vi "UI Selection Valve.vi"(8 "error in":errorcluster) -> (0 "error out":errorcluster)   [LabVIEW 2019, in "Test.lvlib"]
uses:
  Test.lvlib
  Fluidic Process/SubVI/Fluidic Para.ctl
  <vilib>/Utility/file.llb/Read Delimited Spreadsheet (string).vi
  Controller/Controller.lvlib
  Queues/Queues.lvlib
  Fluidic Process/Fluidic Process.lvlib
panel:
  in  "Purge":bool
  in  "Flow Rate":bool
  in  "Stop Process":bool
  out "Remaining Time(s)":dbl
  out "Total Process":string
  out "Current Process":string
  out "Gauge":dbl(knob)=1.2869315802184793e-48 scale=0.0..100.0
  in  "Selection Valve Hold Pressure":bool
  in  "Chip Hold Pressure":bool
  in  "Back":bool
  # "/"
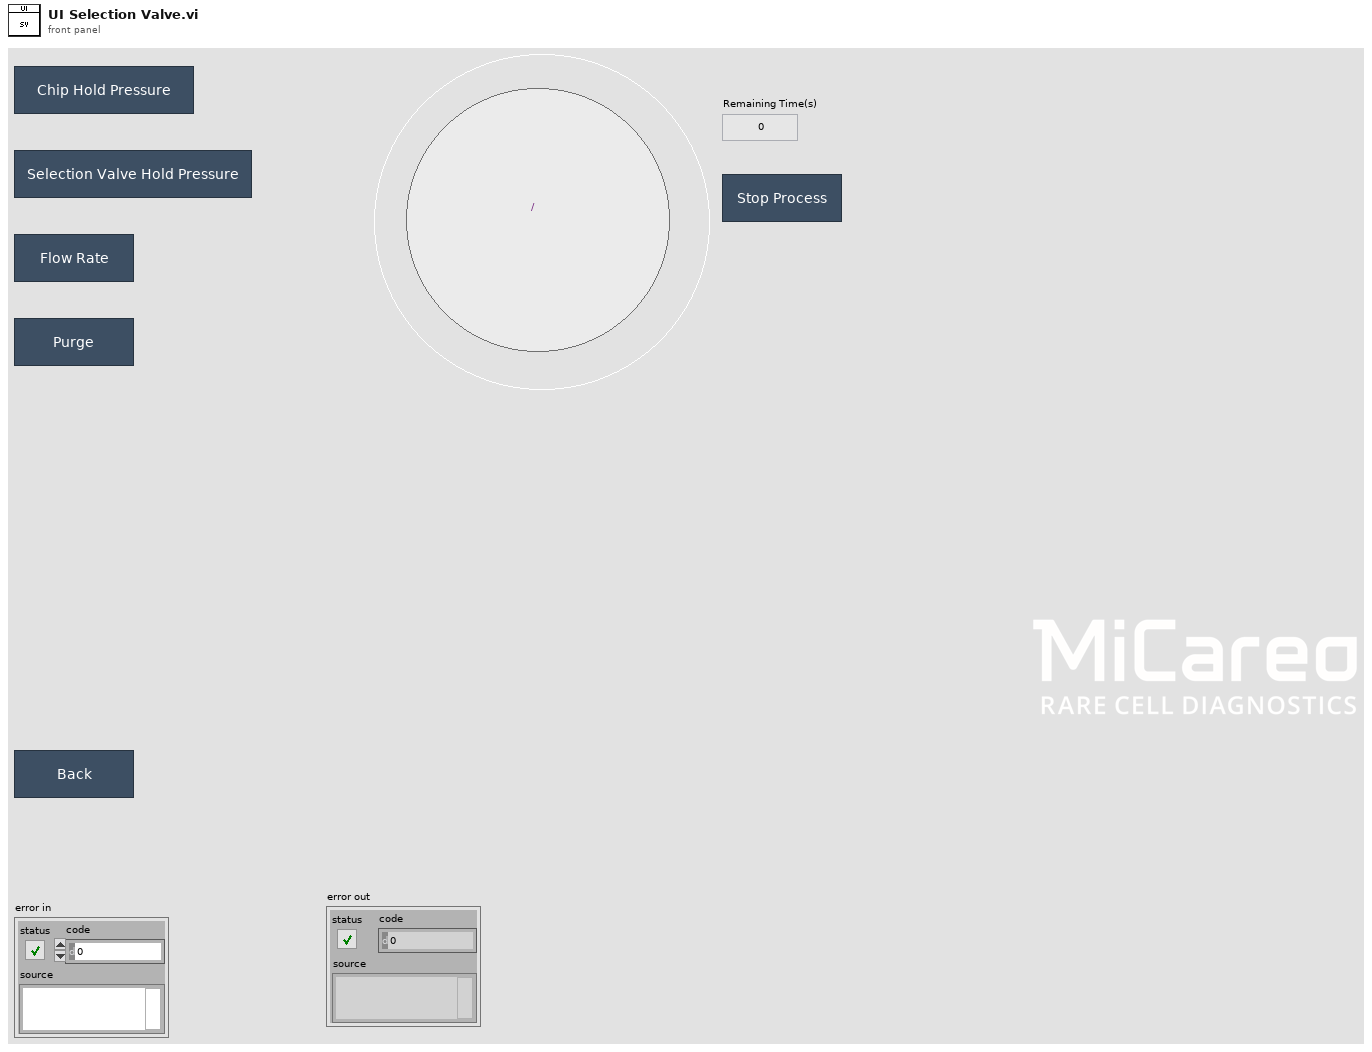
[diagram p1: front panel]
types:
  T1 = enum8{"Enabled", "Disabled", "Disabled and Grayed Out"}
  T2 = typedef "Fluidic Process.lvlib/Fluidic Para.ctl" = cluster{"Read Force Sensor":i32, "Read Regulator":i32, "Read Force Sensor?":bool, "Read Regulator?":bool, "Read Syringe Pump":i32, "Read Syringe Pump?":bool}
  T3 = typedef "Fluidic Process.lvlib/SEQ Data.ctl" = cluster{"Fluidic Process Done?":bool, "Current Process":i32, "Remaining Time":dbl, "Total Process":i32, "Air Sealing":bool, "Force Condition":bool}
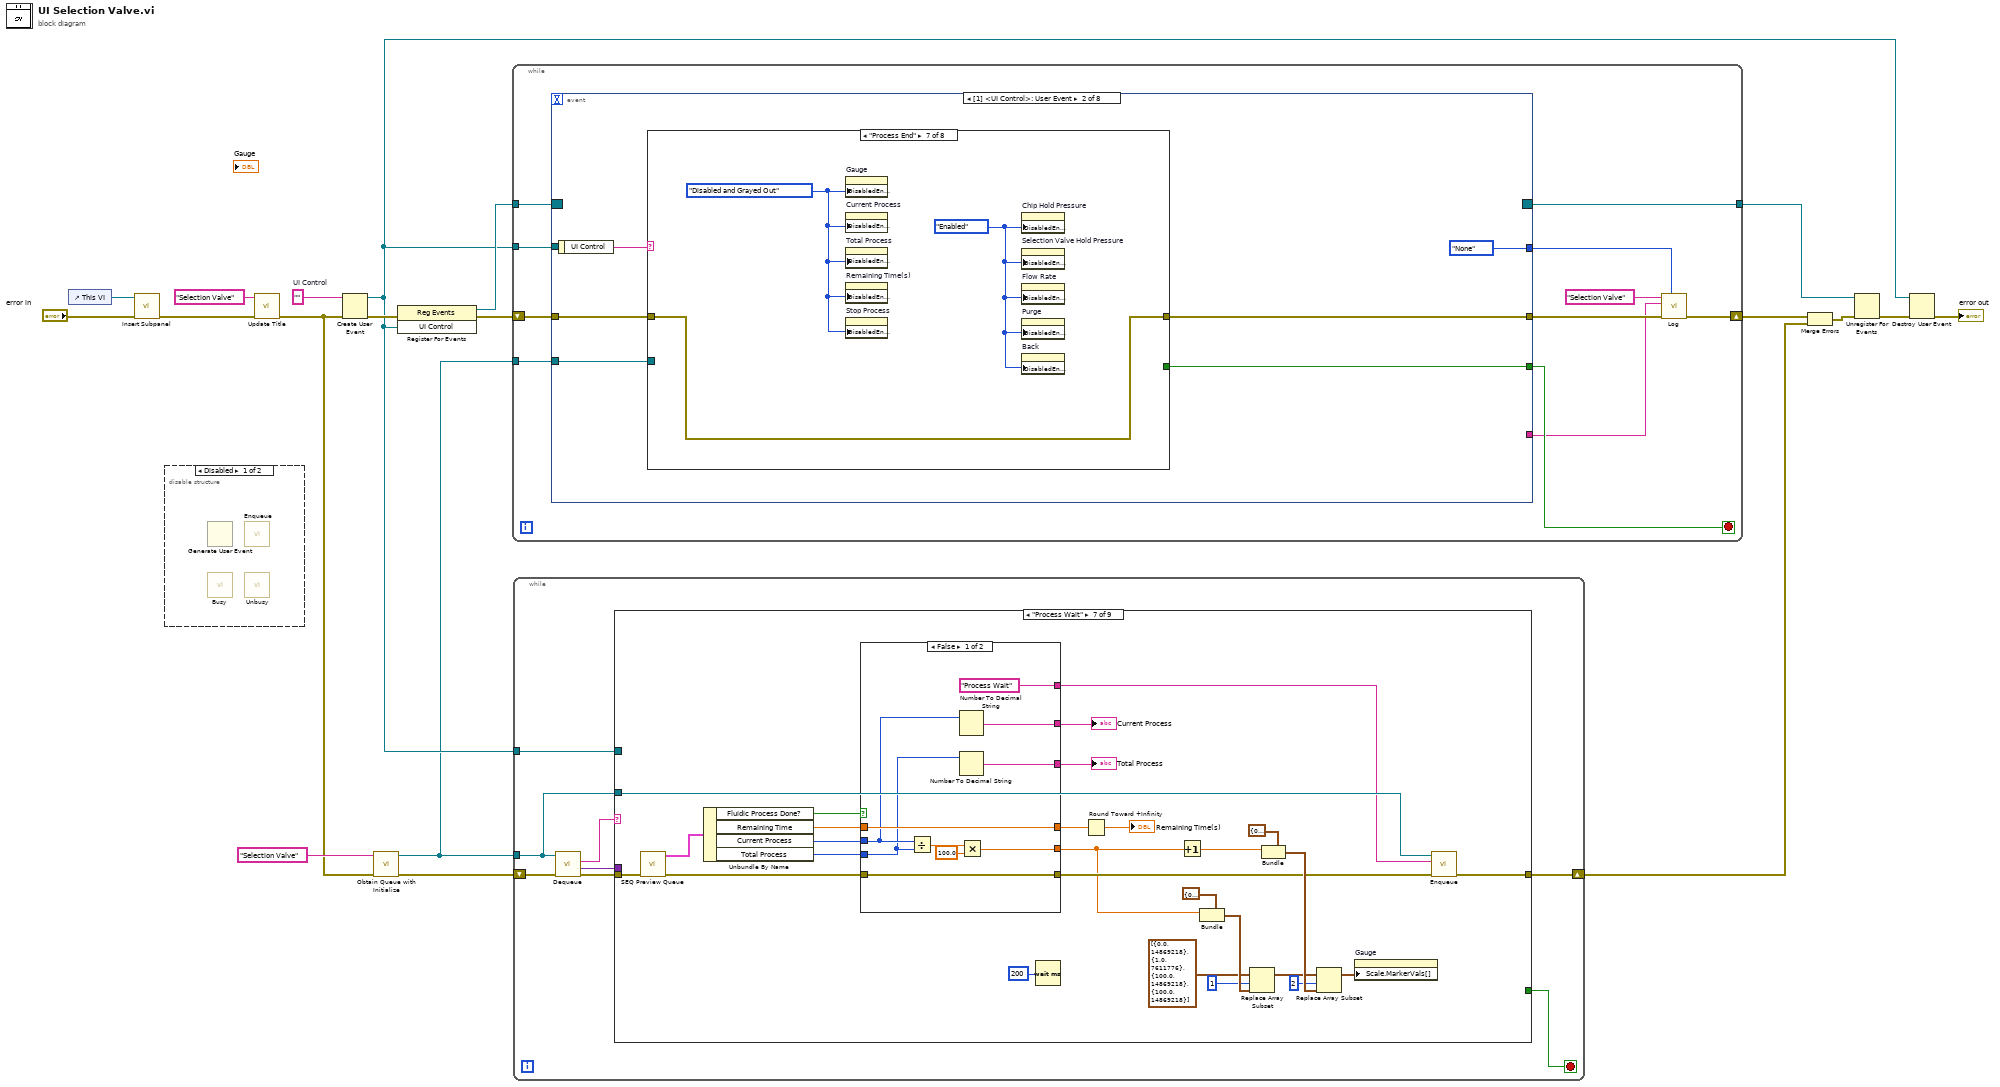
[diagram p0: block diagram]
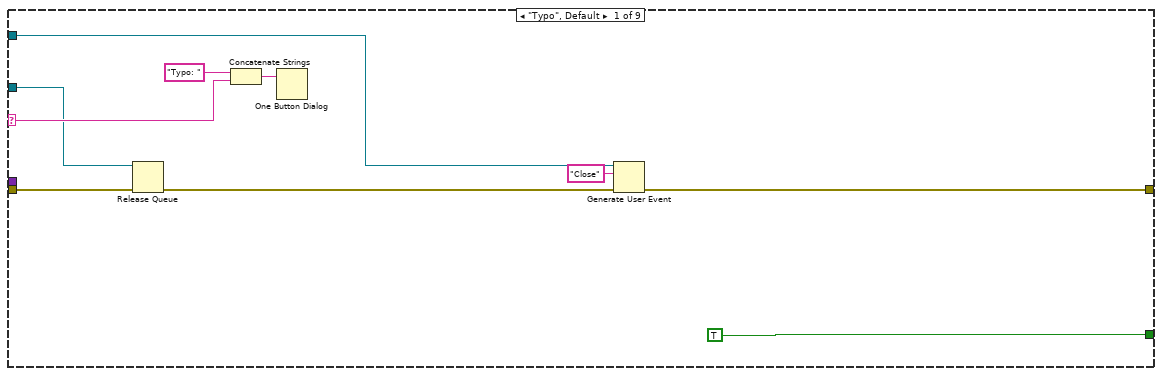
[diagram p3: hidden frame]
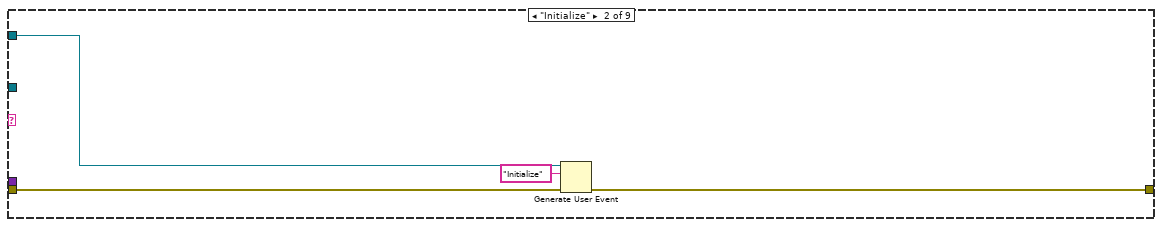
[diagram p4: hidden frame]
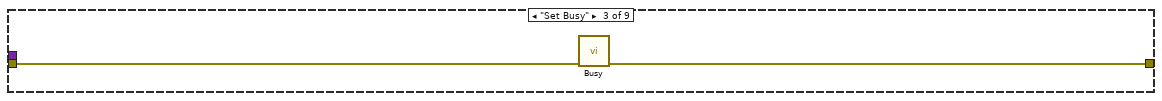
[diagram p5: hidden frame]
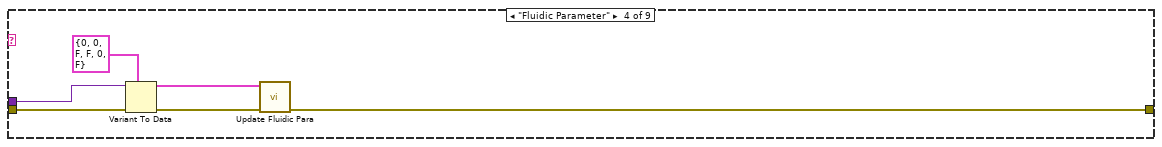
[diagram p6: hidden frame]
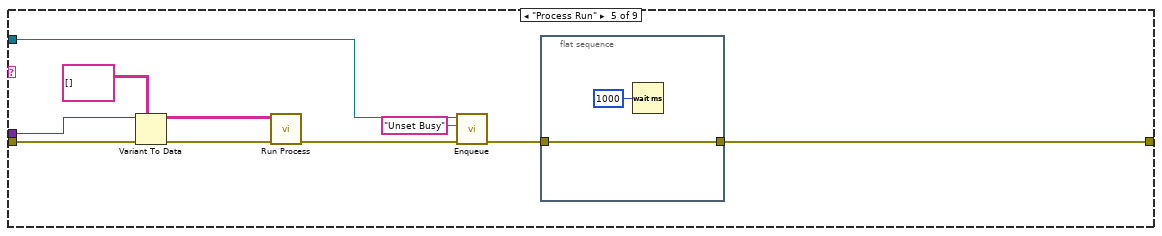
[diagram p7: hidden frame]
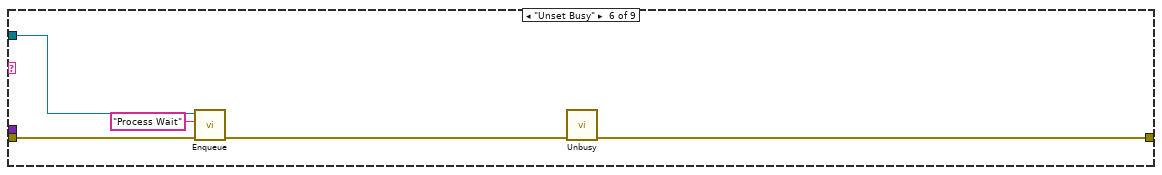
[diagram p8: hidden frame]
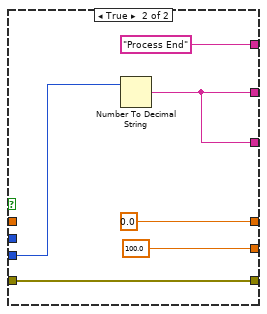
[diagram p9: hidden frame]
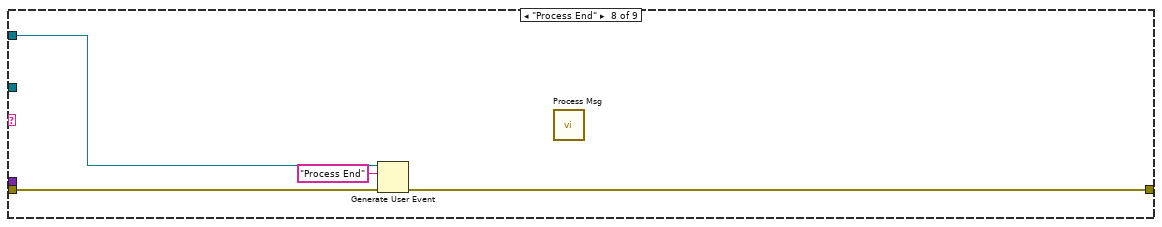
[diagram p10: hidden frame]
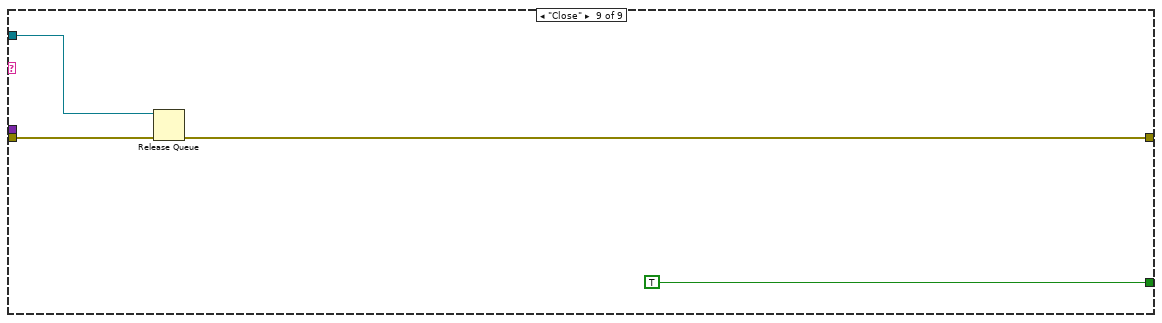
[diagram p11: hidden frame]
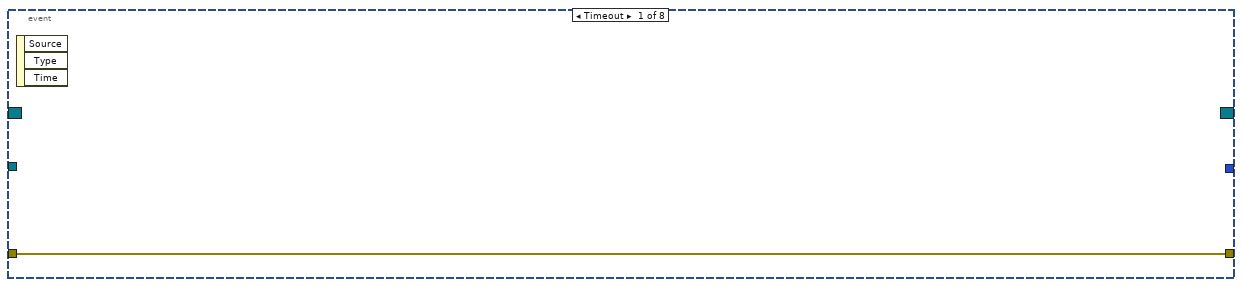
[diagram p12: hidden frame]
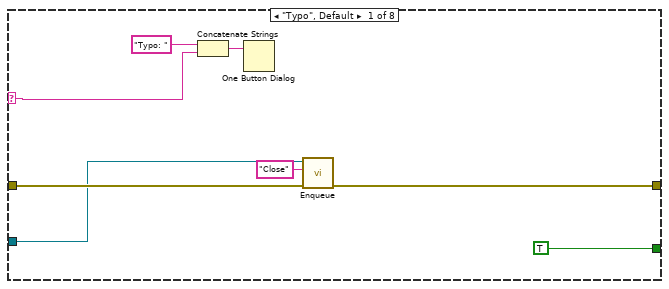
[diagram p13: hidden frame]
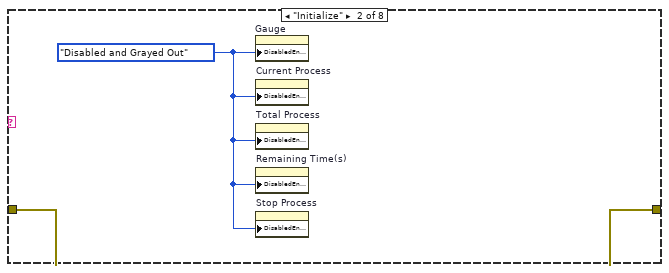
[diagram p14: hidden frame]
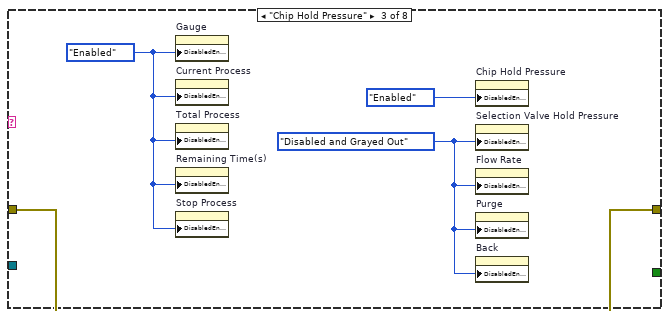
[diagram p15: hidden frame]
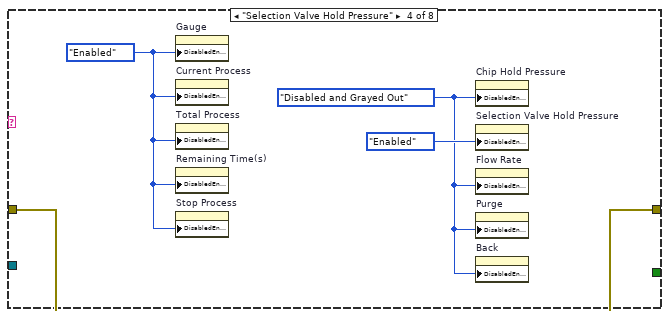
[diagram p16: hidden frame]
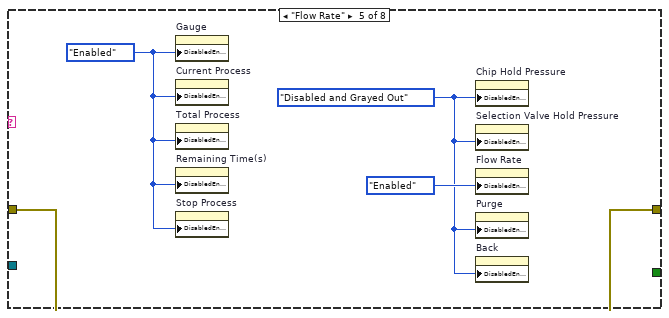
[diagram p17: hidden frame]
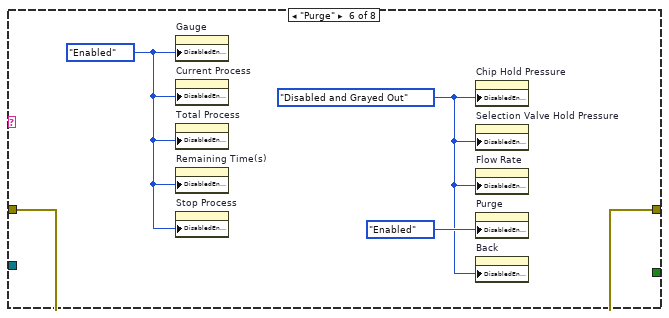
[diagram p18: hidden frame]
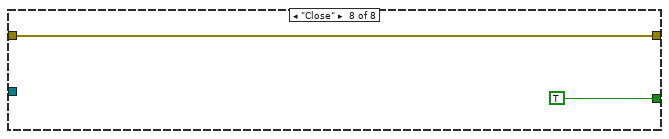
[diagram p19: hidden frame]
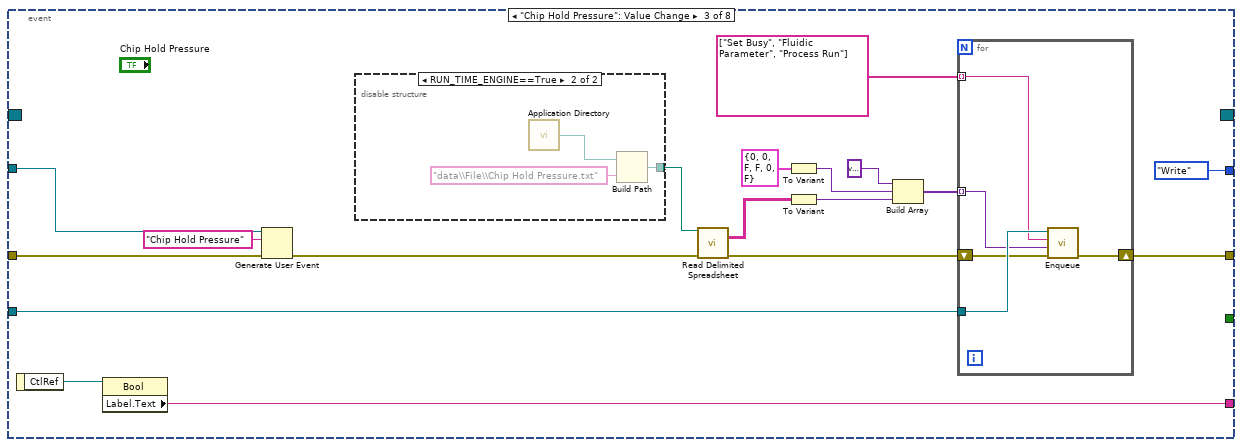
[diagram p20: hidden frame]
diagram:
  w9 = ""  # UI Control
  n1 = control-ref of="This VI"() -> (w8:refnum<vi>)
  n2 = call "Insert Subpanel.vi"("Error In"="error in", "VI Refnum"=w8) -> ("Error Out"=w3:errorcluster)  [unwired: 9 in]
  n3 = disable-structure shown="Disabled" {
    frame Disabled {
      n4 = Generate User Event() -> ()  [unwired: 4 in, 2 out]
      n5 = call "Busy.vi"() -> ()  [unwired: 11 in, 1 out]
      n6 = call "Enqueue.vi"() -> ()  [unwired: 10 in, 2 out]
      n7 = call "Unbusy.vi"() -> ()  [unwired: 11 in, 1 out]
    }
    frame Enabled {
    }
  }
  n8 = call "Update Title.vi"("Error In"=w3, "Title"="Selection Valve") -> ("Error Out"=w2:errorcluster)  [unwired: 9 in]
  n9 = Create User Event(user event datatype=w9, error in=w2) -> (user event=w7:refnum<user-event>, error out=w18:errorcluster)
  n10 = call "Obtain Queue with Initialize.vi"("Error In"=w2, "Queue Name"="Selection Valve") -> ("Error Out"=w6:errorcluster, "Queue out"=w5:refnum<queue>)  [unwired: 8 in]
  n11 = register-events(error in=w18, w7) -> (reference out=w16:refnum<event-registration>, error out=w17:errorcluster)  [unwired: 1 in]
  n12 = while {
    tunnel: w16 -> [w28]
    tunnel: w5 -> [w27]
    shift-right: [w23] -> w14
    shift-left: w17 -> [w30]
    tunnel: [w26] -> w12
    tunnel: w7 -> [w25]
    stop <- w29 stop-if-true
    n13 = event shown="[1] <UI Control>: User Event" {
      selector: w28 -> [_ _ _ _ _ _ _ _]
      dyn-events: [_ _ _ _ _ _ _ _] -> w26
      timeout: _ -> [_ _ _ _ _ _ _ _]
      tunnel: w30 -> [w31 w37 w75 w104 w133 w162 w189 w193]
      tunnel: [_ w33 _ _ _ _ _ TRUE] -> w29
      tunnel: w27 -> [_ w35 w86 w115 w144 w173 _ w195]
      tunnel: [w31 w34 w82 w111 w140 w169 w188 w196] -> w24
      tunnel: w25 -> [_ _ w73 w102 w131 w160 _ _]
      tunnel: [_ enum16{"None", "Write"}."None" ("Action") enum16{"None", "Write"}."Write" ("Action") enum16{"None", "Write"}."Write" ("Action") enum16{"None", "Write"}."Write" ("Action") enum16{"None", "Write"}."Write" ("Action") enum16{"None", "Write"}."Write" ("Action") enum16{"None", "Write"}."Write" ("Action")] -> w21
      tunnel: [_ _ w70 w98 w127 w156 w185 w190] -> w20
      event Timeout {
        n14 = event-data() -> ()  [unwired: 1 in, 3 out]
      }
      event User Event {
        n15 = event-data() -> ("UI Control"=w36:string)  [unwired: 1 in]
        n16 = case shown="\"Process End\"" w36 {
          selector: w36 -> [w40 _ _ _ _ _ _ _]
          tunnel: w37 -> [w45 w47 w51 w55 w59 w63 w66 w68]
          tunnel: w35 -> [w44 _ _ _ _ _ _ _]
          tunnel: [w39 w47 w51 w55 w59 w63 w66 w68] -> w34
          tunnel: [TRUE _ _ _ _ _ _ TRUE] -> w33
          frame "Typo", Default {
            n17 = Concatenate Strings("Typo: " ("string"), w40) -> (w41:string)
            n18 = One Button Dialog(message=w41) -> ()  [unwired: 1 in, 1 out]
            n19 = call "Enqueue.vi"("Error In"=w45, "State"="Close", "Queue in"=w44) -> ("Error Out"=w39:errorcluster)  [unwired: 7 in, 1 out]
          }
          frame "Initialize" {
            w46 = T1."Disabled and Grayed Out" ("Disabled")
            n20 = property on="Gauge" class="Knob (strict)"("DisabledEnum"=w46) -> ()  [unwired: 2 in, 2 out]
            n21 = property on="Current Process" class="Str"("DisabledEnum"=w46) -> ()  [unwired: 2 in, 2 out]
            n22 = property on="Total Process" class="Str"("DisabledEnum"=w46) -> ()  [unwired: 2 in, 2 out]
            n23 = property on="Remaining Time(s)" class="DigNum (strict)"("DisabledEnum"=w46) -> ()  [unwired: 2 in, 2 out]
            n24 = property on="Stop Process" class="Bool"("DisabledEnum"=w46) -> ()  [unwired: 2 in, 2 out]
          }
          frame "Chip Hold Pressure" {
            w49 = T1."Enabled" ("Disabled")
            w48 = T1."Disabled and Grayed Out" ("Disabled")
            n25 = property on="Gauge" class="Knob (strict)"("DisabledEnum"=w49) -> ()  [unwired: 2 in, 2 out]
            n26 = property on="Current Process" class="Str"("DisabledEnum"=w49) -> ()  [unwired: 2 in, 2 out]
            n27 = property on="Total Process" class="Str"("DisabledEnum"=w49) -> ()  [unwired: 2 in, 2 out]
            n28 = property on="Remaining Time(s)" class="DigNum (strict)"("DisabledEnum"=w49) -> ()  [unwired: 2 in, 2 out]
            n29 = property on="Stop Process" class="Bool"("DisabledEnum"=w49) -> ()  [unwired: 2 in, 2 out]
            n30 = property on="Chip Hold Pressure" class="Bool"("DisabledEnum"=T1."Enabled" ("Disabled")) -> ()  [unwired: 2 in, 2 out]
            n31 = property on="Selection Valve Hold Pressure" class="Bool"("DisabledEnum"=w48) -> ()  [unwired: 2 in, 2 out]
            n32 = property on="Flow Rate" class="Bool"("DisabledEnum"=w48) -> ()  [unwired: 2 in, 2 out]
            n33 = property on="Purge" class="Bool"("DisabledEnum"=w48) -> ()  [unwired: 2 in, 2 out]
            n34 = property on="Back" class="Bool"("DisabledEnum"=w48) -> ()  [unwired: 2 in, 2 out]
          }
          frame "Selection Valve Hold Pressure" {
            w54 = T1."Enabled" ("Disabled")
            w52 = T1."Disabled and Grayed Out" ("Disabled")
            n35 = property on="Gauge" class="Knob (strict)"("DisabledEnum"=w54) -> ()  [unwired: 2 in, 2 out]
            n36 = property on="Current Process" class="Str"("DisabledEnum"=w54) -> ()  [unwired: 2 in, 2 out]
            n37 = property on="Total Process" class="Str"("DisabledEnum"=w54) -> ()  [unwired: 2 in, 2 out]
            n38 = property on="Remaining Time(s)" class="DigNum (strict)"("DisabledEnum"=w54) -> ()  [unwired: 2 in, 2 out]
            n39 = property on="Stop Process" class="Bool"("DisabledEnum"=w54) -> ()  [unwired: 2 in, 2 out]
            n40 = property on="Chip Hold Pressure" class="Bool"("DisabledEnum"=w52) -> ()  [unwired: 2 in, 2 out]
            n41 = property on="Selection Valve Hold Pressure" class="Bool"("DisabledEnum"=T1."Enabled" ("Disabled")) -> ()  [unwired: 2 in, 2 out]
            n42 = property on="Flow Rate" class="Bool"("DisabledEnum"=w52) -> ()  [unwired: 2 in, 2 out]
            n43 = property on="Purge" class="Bool"("DisabledEnum"=w52) -> ()  [unwired: 2 in, 2 out]
            n44 = property on="Back" class="Bool"("DisabledEnum"=w52) -> ()  [unwired: 2 in, 2 out]
          }
          frame "Flow Rate" {
            w58 = T1."Enabled" ("Disabled")
            w56 = T1."Disabled and Grayed Out" ("Disabled")
            n45 = property on="Gauge" class="Knob (strict)"("DisabledEnum"=w58) -> ()  [unwired: 2 in, 2 out]
            n46 = property on="Current Process" class="Str"("DisabledEnum"=w58) -> ()  [unwired: 2 in, 2 out]
            n47 = property on="Total Process" class="Str"("DisabledEnum"=w58) -> ()  [unwired: 2 in, 2 out]
            n48 = property on="Remaining Time(s)" class="DigNum (strict)"("DisabledEnum"=w58) -> ()  [unwired: 2 in, 2 out]
            n49 = property on="Stop Process" class="Bool"("DisabledEnum"=w58) -> ()  [unwired: 2 in, 2 out]
            n50 = property on="Chip Hold Pressure" class="Bool"("DisabledEnum"=w56) -> ()  [unwired: 2 in, 2 out]
            n51 = property on="Selection Valve Hold Pressure" class="Bool"("DisabledEnum"=w56) -> ()  [unwired: 2 in, 2 out]
            n52 = property on="Flow Rate" class="Bool"("DisabledEnum"=T1."Enabled" ("Disabled")) -> ()  [unwired: 2 in, 2 out]
            n53 = property on="Purge" class="Bool"("DisabledEnum"=w56) -> ()  [unwired: 2 in, 2 out]
            n54 = property on="Back" class="Bool"("DisabledEnum"=w56) -> ()  [unwired: 2 in, 2 out]
          }
          frame "Purge" {
            w62 = T1."Enabled" ("Disabled")
            w60 = T1."Disabled and Grayed Out" ("Disabled")
            n55 = property on="Gauge" class="Knob (strict)"("DisabledEnum"=w62) -> ()  [unwired: 2 in, 2 out]
            n56 = property on="Current Process" class="Str"("DisabledEnum"=w62) -> ()  [unwired: 2 in, 2 out]
            n57 = property on="Total Process" class="Str"("DisabledEnum"=w62) -> ()  [unwired: 2 in, 2 out]
            n58 = property on="Remaining Time(s)" class="DigNum (strict)"("DisabledEnum"=w62) -> ()  [unwired: 2 in, 2 out]
            n59 = property on="Stop Process" class="Bool"("DisabledEnum"=w62) -> ()  [unwired: 2 in, 2 out]
            n60 = property on="Chip Hold Pressure" class="Bool"("DisabledEnum"=w60) -> ()  [unwired: 2 in, 2 out]
            n61 = property on="Selection Valve Hold Pressure" class="Bool"("DisabledEnum"=w60) -> ()  [unwired: 2 in, 2 out]
            n62 = property on="Flow Rate" class="Bool"("DisabledEnum"=w60) -> ()  [unwired: 2 in, 2 out]
            n63 = property on="Purge" class="Bool"("DisabledEnum"=T1."Enabled" ("Disabled")) -> ()  [unwired: 2 in, 2 out]
            n64 = property on="Back" class="Bool"("DisabledEnum"=w60) -> ()  [unwired: 2 in, 2 out]
          }
          frame "Process End" {
            w65 = T1."Disabled and Grayed Out" ("Disabled")
            w64 = T1."Enabled" ("Disabled")
            n65 = property on="Gauge" class="Knob (strict)"("DisabledEnum"=w65) -> ()  [unwired: 2 in, 2 out]
            n66 = property on="Current Process" class="Str"("DisabledEnum"=w65) -> ()  [unwired: 2 in, 2 out]
            n67 = property on="Total Process" class="Str"("DisabledEnum"=w65) -> ()  [unwired: 2 in, 2 out]
            n68 = property on="Remaining Time(s)" class="DigNum (strict)"("DisabledEnum"=w65) -> ()  [unwired: 2 in, 2 out]
            n69 = property on="Stop Process" class="Bool"("DisabledEnum"=w65) -> ()  [unwired: 2 in, 2 out]
            n70 = property on="Chip Hold Pressure" class="Bool"("DisabledEnum"=w64) -> ()  [unwired: 2 in, 2 out]
            n71 = property on="Selection Valve Hold Pressure" class="Bool"("DisabledEnum"=w64) -> ()  [unwired: 2 in, 2 out]
            n72 = property on="Flow Rate" class="Bool"("DisabledEnum"=w64) -> ()  [unwired: 2 in, 2 out]
            n73 = property on="Purge" class="Bool"("DisabledEnum"=w64) -> ()  [unwired: 2 in, 2 out]
            n74 = property on="Back" class="Bool"("DisabledEnum"=w64) -> ()  [unwired: 2 in, 2 out]
          }
          frame "Close" {
          }
        }
      }
      event "Chip Hold Pressure": Value Change {
        n75 = event-data() -> ("CtlRef"=w71:refnum<vi>)  [unwired: 1 in]
        n76 = property class="Bool"(reference=w71) -> ("Label.Text"=w70:string)  [unwired: 1 in, 2 out]
        n77 = Generate User Event(user event=w73, event data cluster="Chip Hold Pressure" ("event data"), error in=w75) -> (error out=w74:errorcluster)  [unwired: 1 in, 1 out]
        n78 = disable-structure shown="RUN_TIME_ENGINE==True" {
          disable-tunnel: [w87 w90] -> w84
          frame condition #0 (active) {
            n79 = call <vilib>:"Application Directory.vi"() -> ("Application Directory"=w89:path)
            n80 = Build Path(base path=w89, name or relative path="Fluidic Process\\File\\Chip Hold Pressure.txt") -> (appended path=w87:path)
          }
          frame condition #1 {
            n81 = call <vilib>:"Application Directory.vi"() -> ("Application Directory"=w92:path)
            n82 = Build Path(base path=w92, name or relative path="data\\File\\Chip Hold Pressure.txt") -> (appended path=w90:path)
          }
        }
        n83 = call-poly <vilib>:"Read Delimited Spreadsheet.vi"("file path (dialog if empty)"=w84, "error in (no error)"=w74) -> ("all rows"=w83:string[][], "error out"=w85:errorcluster)  [unwired: 8 in, 4 out]
        n84 = To Variant(anything=T2 {"Read Force Sensor"=0, "Read Regulator"=0, "Read Force Sensor?"=FALSE, "Read Regulator?"=FALSE, "Read Syringe Pump"=0, "Read Syringe Pump?"=FALSE} ("Cluster")) -> (Variant=w78:variant)
        n85 = To Variant(anything=w83) -> (Variant=w80:variant)
        n86 = Build Array(variant, w78, w80) -> (w77:variant[])
        n87 = for {
          tunnel: w86 -> [w97]
          shift-right: [w95] -> w82
          shift-left: w85 -> [w96]
          tunnel: string[] ["Set Busy", "Fluidic Parameter", "Process Run"] -> [w94] mode=indexing
          tunnel: w77 -> [w93] mode=indexing
          n88 = call "Enqueue.vi"("Error In"=w96, "Data"=w93, "State"=w94, "Queue in"=w97) -> ("Error Out"=w95:errorcluster)  [unwired: 6 in, 1 out]
        }
      }
      event "Selection Valve Hold Pressure": Value Change {
        n89 = event-data() -> ("CtlRef"=w99:refnum<vi>)  [unwired: 1 in]
        n90 = property class="Bool"(reference=w99) -> ("Label.Text"=w98:string)  [unwired: 1 in, 2 out]
        n91 = Generate User Event(user event=w102, event data cluster="Selection Valve Hold Pressure" ("event data"), error in=w104) -> (error out=w103:errorcluster)  [unwired: 1 in, 1 out]
        n92 = disable-structure shown="RUN_TIME_ENGINE==False, Default" {
          disable-tunnel: [w116 w119] -> w113
          frame condition #0 (active) {
            n93 = call <vilib>:"Application Directory.vi"() -> ("Application Directory"=w118:path)
            n94 = Build Path(base path=w118, name or relative path="Fluidic Process\\File\\Selection Valve Hold Pressure.txt") -> (appended path=w116:path)
          }
          frame condition #1 {
            n95 = call <vilib>:"Application Directory.vi"() -> ("Application Directory"=w121:path)
            n96 = Build Path(base path=w121, name or relative path="data\\File\\Selection Valve Hold Pressure.txt") -> (appended path=w119:path)
          }
        }
        n97 = call-poly <vilib>:"Read Delimited Spreadsheet.vi"("file path (dialog if empty)"=w113, "error in (no error)"=w103) -> ("all rows"=w112:string[][], "error out"=w114:errorcluster)  [unwired: 8 in, 4 out]
        n98 = To Variant(anything=T2 {"Read Force Sensor"=0, "Read Regulator"=0, "Read Force Sensor?"=FALSE, "Read Regulator?"=FALSE, "Read Syringe Pump"=0, "Read Syringe Pump?"=FALSE} ("Cluster")) -> (Variant=w107:variant)
        n99 = To Variant(anything=w112) -> (Variant=w109:variant)
        n100 = Build Array(variant, w107, w109) -> (w106:variant[])
        n101 = for {
          tunnel: w115 -> [w126]
          shift-right: [w124] -> w111
          shift-left: w114 -> [w125]
          tunnel: string[] ["Set Busy", "Fluidic Parameter", "Process Run"] -> [w123] mode=indexing
          tunnel: w106 -> [w122] mode=indexing
          n102 = call "Enqueue.vi"("Error In"=w125, "Data"=w122, "State"=w123, "Queue in"=w126) -> ("Error Out"=w124:errorcluster)  [unwired: 6 in, 1 out]
        }
      }
      event "Flow Rate": Value Change {
        n103 = event-data() -> ("CtlRef"=w128:refnum<vi>)  [unwired: 1 in]
        n104 = property class="Bool"(reference=w128) -> ("Label.Text"=w127:string)  [unwired: 1 in, 2 out]
        n105 = Generate User Event(user event=w131, event data cluster="Flow Rate" ("event data"), error in=w133) -> (error out=w132:errorcluster)  [unwired: 1 in, 1 out]
        n106 = disable-structure shown="RUN_TIME_ENGINE==True" {
          disable-tunnel: [w145 w148] -> w142
          frame condition #0 (active) {
            n107 = call <vilib>:"Application Directory.vi"() -> ("Application Directory"=w147:path)
            n108 = Build Path(base path=w147, name or relative path="Fluidic Process\\File\\Flow Rate.txt") -> (appended path=w145:path)
          }
          frame condition #1 {
            n109 = call <vilib>:"Application Directory.vi"() -> ("Application Directory"=w150:path)
            n110 = Build Path(base path=w150, name or relative path="data\\File\\Flow Rate.txt") -> (appended path=w148:path)
          }
        }
        n111 = call-poly <vilib>:"Read Delimited Spreadsheet.vi"("file path (dialog if empty)"=w142, "error in (no error)"=w132) -> ("all rows"=w141:string[][], "error out"=w143:errorcluster)  [unwired: 8 in, 4 out]
        n112 = To Variant(anything=T2 {"Read Force Sensor"=0, "Read Regulator"=0, "Read Force Sensor?"=FALSE, "Read Regulator?"=FALSE, "Read Syringe Pump"=0, "Read Syringe Pump?"=FALSE} ("Cluster")) -> (Variant=w136:variant)
        n113 = To Variant(anything=w141) -> (Variant=w138:variant)
        n114 = Build Array(variant, w136, w138) -> (w135:variant[])
        n115 = for {
          tunnel: w144 -> [w155]
          shift-right: [w153] -> w140
          shift-left: w143 -> [w154]
          tunnel: string[] ["Set Busy", "Fluidic Parameter", "Process Run"] -> [w152] mode=indexing
          tunnel: w135 -> [w151] mode=indexing
          n116 = call "Enqueue.vi"("Error In"=w154, "Data"=w151, "State"=w152, "Queue in"=w155) -> ("Error Out"=w153:errorcluster)  [unwired: 6 in, 1 out]
        }
      }
      event "Purge": Value Change {
        n117 = event-data() -> ("CtlRef"=w157:refnum<vi>)  [unwired: 1 in]
        n118 = property class="Bool"(reference=w157) -> ("Label.Text"=w156:string)  [unwired: 1 in, 2 out]
        n119 = Generate User Event(user event=w160, event data cluster="Purge" ("event data"), error in=w162) -> (error out=w161:errorcluster)  [unwired: 1 in, 1 out]
        n120 = disable-structure shown="RUN_TIME_ENGINE==True" {
          disable-tunnel: [w174 w177] -> w171
          frame condition #0 (active) {
            n121 = call <vilib>:"Application Directory.vi"() -> ("Application Directory"=w176:path)
            n122 = Build Path(base path=w176, name or relative path="Fluidic Process\\File\\Purge.txt") -> (appended path=w174:path)
          }
          frame condition #1 {
            n123 = call <vilib>:"Application Directory.vi"() -> ("Application Directory"=w179:path)
            n124 = Build Path(base path=w179, name or relative path="data\\File\\Purge.txt") -> (appended path=w177:path)
          }
        }
        n125 = call-poly <vilib>:"Read Delimited Spreadsheet.vi"("file path (dialog if empty)"=w171, "error in (no error)"=w161) -> ("all rows"=w170:string[][], "error out"=w172:errorcluster)  [unwired: 8 in, 4 out]
        n126 = To Variant(anything=T2 {"Read Force Sensor"=0, "Read Regulator"=0, "Read Force Sensor?"=FALSE, "Read Regulator?"=FALSE, "Read Syringe Pump"=3, "Read Syringe Pump?"=TRUE} ("Cluster")) -> (Variant=w165:variant)
        n127 = To Variant(anything=w170) -> (Variant=w167:variant)
        n128 = Build Array(variant, w165, w167) -> (w164:variant[])
        n129 = for {
          tunnel: w173 -> [w184]
          shift-right: [w182] -> w169
          shift-left: w172 -> [w183]
          tunnel: string[] ["Set Busy", "Fluidic Parameter", "Process Run"] -> [w181] mode=indexing
          tunnel: w164 -> [w180] mode=indexing
          n130 = call "Enqueue.vi"("Error In"=w183, "Data"=w180, "State"=w181, "Queue in"=w184) -> ("Error Out"=w182:errorcluster)  [unwired: 6 in, 1 out]
        }
      }
      event "Stop Process": Value Change {
        n131 = event-data() -> ("CtlRef"=w186:refnum<vi>)  [unwired: 1 in]
        n132 = property class="Bool"(reference=w186) -> ("Label.Text"=w185:string)  [unwired: 1 in, 2 out]
        n133 = call "Stop Process.vi"("Error In"=w189) -> ("Error Out"=w188:errorcluster)  [unwired: 10 in]
      }
      event "Back": Value Change {
        n134 = event-data() -> ("CtlRef"=w191:refnum<vi>)  [unwired: 1 in]
        n135 = property class="Bool"(reference=w191) -> ("Label.Text"=w190:string)  [unwired: 1 in, 2 out]
        n136 = call "Enqueue.vi"("Error In"=w193, "State"="Close", "Queue in"=w195) -> ("Error Out"=w196:errorcluster)  [unwired: 7 in, 1 out]
      }
    }
    n137 = call "Log.vi"("Action"=w21, "error in"=w24, "State"=w20, "Page Name"="Selection Valve") -> ("error out"=w23:errorcluster)  [unwired: 7 in]
  }
  n138 = while {
    tunnel: w5 -> [w202]
    shift-right: [w200] -> w13
    shift-left: w6 -> [w205]
    tunnel: w7 -> [w199]
    stop <- w198 stop-if-true
    n139 = call "Dequeue.vi"("Error In"=w205, "Queue in"=w202) -> ("Error Out"=w201:errorcluster, "Data"=w203:variant, "State"=w204:string)  [unwired: 6 in, 1 out]
    n140 = case shown="\"Process Wait\"" w204 {
      selector: w204 -> [w213 _ _ _ _ _ _ _ _]
      tunnel: w203 -> [_ _ _ w226 w236 _ _ _ _]
      tunnel: w202 -> [w206 _ _ _ w231 w243 w249 _ w293]
      tunnel: w201 -> [w208 w219 w221 w227 w237 w244 w271 w291 w295]
      tunnel: [TRUE _ _ _ _ _ _ _ TRUE] -> w198
      tunnel: [w211 w218 w220 w222 w228 w240 w255 w290 w294] -> w200
      tunnel: w199 -> [w210 w217 _ _ _ _ _ w289 _]
      frame "Typo", Default {
        n141 = Release Queue(queue=w206, error in (no error)=w208) -> (error out=w207:errorcluster)  [unwired: 1 in, 2 out]
        n142 = Concatenate Strings("Typo: " ("string"), w213) -> (w215:string)
        n143 = One Button Dialog(message=w215) -> ()  [unwired: 1 in, 1 out]
        n144 = Generate User Event(user event=w210, event data cluster="Close" ("event data"), error in=w207) -> (error out=w211:errorcluster)  [unwired: 1 in, 1 out]
      }
      frame "Initialize" {
        n145 = Generate User Event(user event=w217, event data cluster="Initialize" ("event data"), error in=w219) -> (error out=w218:errorcluster)  [unwired: 1 in, 1 out]
      }
      frame "Set Busy" {
        n146 = call "Busy.vi"("Error In"=w221) -> ("Error Out"=w220:errorcluster)  [unwired: 10 in]
      }
      frame "Fluidic Parameter" {
        n147 = Variant To Data(error in=w227, type=T2 {"Read Force Sensor"=0, "Read Regulator"=0, "Read Force Sensor?"=FALSE, "Read Regulator?"=FALSE, "Read Syringe Pump"=0, "Read Syringe Pump?"=FALSE} ("Cluster"), Variant=w226) -> (data=w223:T2, error out=w224:errorcluster)
        n148 = call "Update Fluidic Para.vi"("Error In"=w224, "Fluidic Para"=w223) -> ("Error Out"=w222:errorcluster)  [unwired: 9 in]
      }
      frame "Process Run" {
        n149 = Variant To Data(error in=w237, type=string[][] [] ("all rows"), Variant=w236) -> (data=w233:string[][], error out=w234:errorcluster)
        n150 = call "Run Process.vi"("Error In"=w234, "Fluidic Process in"=w233) -> ("Error Out"=w232:errorcluster)  [unwired: 9 in]
        n151 = call "Enqueue.vi"("Error In"=w232, "State"="Unset Busy", "Queue in"=w231) -> ("Error Out"=w229:errorcluster)  [unwired: 7 in, 1 out]
        n152 = flat-sequence {
          tunnel: w229 -> [w239]
          tunnel: [w239] -> w228
          frame #0 {
            n153 = Wait (ms)(milliseconds to wait=u32 1000) -> ()  [unwired: 1 out]
          }
        }
      }
      frame "Unset Busy" {
        n154 = call "Enqueue.vi"("Error In"=w244, "State"="Process Wait", "Queue in"=w243) -> ("Error Out"=w241:errorcluster)  [unwired: 7 in, 1 out]
        n155 = call "Unbusy.vi"("Error In"=w241) -> ("Error Out"=w240:errorcluster)  [unwired: 10 in]
      }
      frame "Process Wait" {
        n156 = call "SEQ Preview Queue.vi"("error in"=w271) -> ("error out"=w268:errorcluster, "SEQ Data"=w270:T3)  [unwired: 9 in]
        n157 = Unbundle By Name(w270) -> ("Fluidic Process Done?"=w269:bool, "Remaining Time"=w254:dbl, "Current Process"=w253:i32, "Total Process"=w252:i32)
        n158 = case shown="False" w269 {
          tunnel: w268 -> [w279 w287]
          tunnel: [w279 w287] -> w256
          tunnel: w254 -> [w278 _]
          tunnel: w253 -> [w276 _]
          tunnel: w252 -> [w275 w286]
          tunnel: [w278 0.0 ("Remaining Time")] -> w250
          tunnel: [w277 100.0] -> w251
          tunnel: [w274 w285] -> w248
          tunnel: [w273 w285] -> w247
          tunnel: ["Process Wait" "Process End"] -> w246
          frame False {
            n159 = Divide(x=w276, y=w275) -> (x/y=w281:dbl)
            n160 = Number To Decimal String(number=w276) -> (decimal integer string=w274:string)  [unwired: 1 in]
            n161 = Number To Decimal String(number=w275) -> (decimal integer string=w273:string)  [unwired: 1 in]
            n162 = Multiply(x=w281, y=100.0) -> (x*y=w277:dbl)
          }
          frame True {
            n163 = Number To Decimal String(number=w286) -> (decimal integer string=w285:string)  [unwired: 1 in]
          }
        }
        "Total Process" <- w247
        "Current Process" <- w248
        n164 = Wait (ms)(milliseconds to wait=u32 200) -> ()  [unwired: 1 out]
        n165 = Round Toward +Infinity(x=w250) -> (ceil(x): smallest int >= x=→"Remaining Time(s)":dbl)
        n166 = Increment(x=w251) -> (x+1=w264:dbl)
        n167 = Bundle(cluster=cluster{dbl, i32} {0.0, 7611776}, w251) -> (w263:cluster{dbl, i32})  [unwired: 1 in]
        n168 = Replace Array Subset(array=cluster{dbl, u32}[] [{0.0, 14869218}, {1.0, 7611776}, {100.0, 14869218}, {100.0, 14869218}] ("Scale.Marker Values[]"), new element=w263, index=1) -> (w265:cluster{dbl, u32}[])
        n169 = Bundle(cluster=cluster{dbl, i32} {0.0, 14869218}, w264) -> (w266:cluster{dbl, i32})  [unwired: 1 in]
        n170 = Replace Array Subset(array=w265, new element=w266, index=2) -> (w267:cluster{dbl, u32}[])
        n171 = property on="Gauge" class="Knob (strict)"("Scale.MarkerVals[]"=w267) -> ()  [unwired: 2 in, 2 out]
        n172 = call "Enqueue.vi"("Error In"=w256, "State"=w246, "Queue in"=w249) -> ("Error Out"=w255:errorcluster)  [unwired: 7 in, 1 out]
      }
      frame "Process End" {
        n173 = Generate User Event(user event=w289, event data cluster="Process End" ("event data"), error in=w291) -> (error out=w290:errorcluster)  [unwired: 1 in, 1 out]
        n174 = call "Process Msg"() -> ()  [unwired: 10 in, 2 out]
      }
      frame "Close" {
        n175 = Release Queue(queue=w293, error in (no error)=w295) -> (error out=w294:errorcluster)  [unwired: 1 in, 2 out]
      }
    }
  }
  n176 = Merge Errors(w14, w13) -> (w11:errorcluster)
  n177 = Unregister For Events(event registration refnum=w12, error in=w11) -> (error out=w10:errorcluster)
  n178 = Destroy User Event(user event=w7, error in=w10) -> (error out=→"error out":errorcluster)
